vi "5.0-State Update.vi"(1 "6.0 ForeBrain State In":T1) -> (0 "6.0 ForeBrain State out":T1)   [LabVIEW 2010]
uses:
  3-Midbrain/3.0-Global.vi
  4-High Neurons/4.0-Midbrain State.ctl
  6-OCU Neurons/6.0-Forbrain State.ctl
  5.0-Global.vi
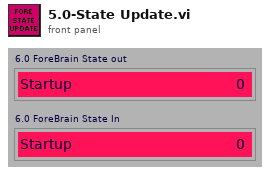
[diagram p1: front panel]
types:
  T1 = typedef "6.0-Forbrain State.ctl" = enum16{"Startup", "Waiting to Run", "Running-OlinOval", "Running-ChannelFollow", "Running-WallFollow", "Running-OpenTransit", "Running-Joystick Training", "Shutdown", "Restart", "New IP"}
  T2 = typedef "4.0-Midbrain State.ctl" = enum16{"Startup", "Waiting to Run", "Running-OlinOval", "Running-ChannelFollow", "Running-WallFollow", "Running-OpenTransit", "Running-Joystick Training", "Shutdown", "Restart", "New IP"}
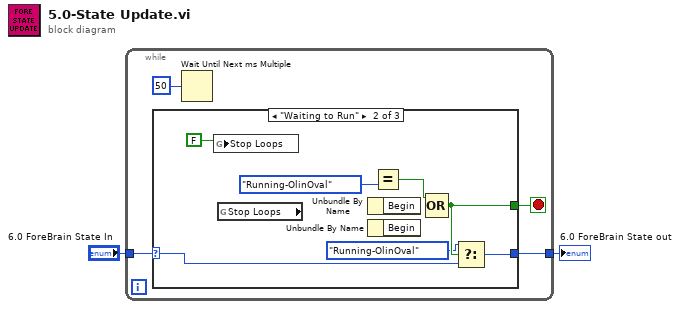
[diagram p0: block diagram]
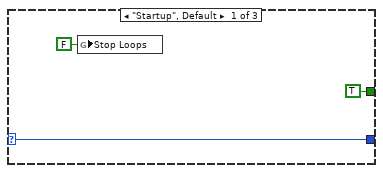
[diagram p2: hidden frame]
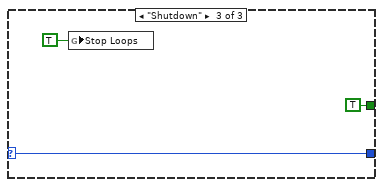
[diagram p3: hidden frame]
diagram:
  n1 = while {
    tunnel: "6.0 ForeBrain State In" -> [w6]
    tunnel: [w5] -> w1
    stop <- w3 stop-if-true
    n2 = case shown="\"Waiting to Run\"" w6 {
      selector: w6 -> [w9 w16 w18]
      tunnel: [w9 w15 w18] -> w5
      tunnel: [TRUE w14 TRUE ("Begin")] -> w3
      frame "Startup", Default {
        n3 = global write "3.0-Global.vi" "Stop Loops"(FALSE ("Stop Loops")) -> ()
      }
      frame "Waiting to Run" {
        n4 = global write "5.0-Global.vi" "Stop Loops"(FALSE ("Stop Loops")) -> ()
        n5 = global read "5.0-Global.vi" "Stop Loops"() -> ()  [unwired: 1 out]
        n6 = Unbundle By Name() -> ()  [unwired: 1 in, 1 out]
        n7 = Unbundle By Name() -> ()  [unwired: 1 in, 1 out]
        n8 = Equal?(y=4.0-Midbrain_State."Running-OlinOval" ("4.0-Midbrain State")) -> (x = y?=w13:bool)  [unwired: 1 in]
        n9 = Compound Arithmetic op=OR(w13) -> (w14:bool)  [unwired: 2 in]
        n10 = Select(t=6.0-Forbrain_State."Running-OlinOval", s=w14, f=w16) -> (s? t:f=w15:T1)
      }
      frame "Shutdown" {
        n11 = global write "3.0-Global.vi" "Stop Loops"(TRUE ("Stop Loops")) -> ()
      }
    }
    n12 = Wait Until Next ms Multiple(millisecond multiple=u32 50) -> ()  [unwired: 1 out]
  }
  "6.0 ForeBrain State out" <- w1
